vi "例10.8  连续采集图像并保存至avi.vi"() -> ()   [LabVIEW 2017]
doc: "The Grab VI acquires images continuously and displays the images in an image control using high-level acquisition VIs. A grab is appropriate for high-speed applications in which you need to process only one image at a time."
uses:
  <vilib>/userdefined/High Color/IMAQdx.ctl
  <vilib>/vision/driver/NI_Vision_Acquisition_Software.lvlib
panel:
  in  "Frames Per Second":u32=30
  in  "Camera Name":T1
  out "Buffer Number":u32
  out "Image":T2(plugin-control)
  in  "stop":bool
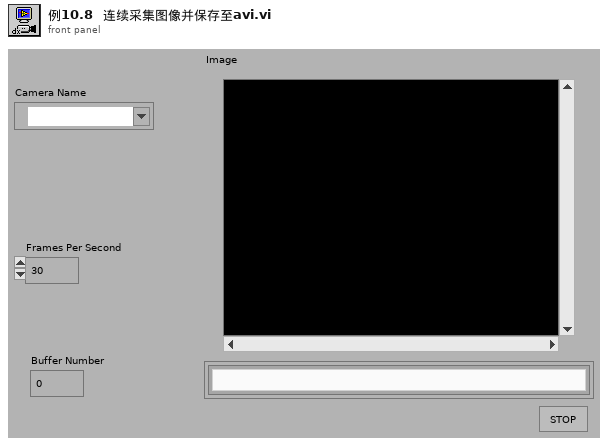
[diagram p1: front panel]
types:
  T1 = typedef "IMAQdx.ctl" = refnum<k21>
  T2 = typedef "IMAQ Image.ctl" = refnum<image>
  T3 = typedef "AviRefnum.ctl" = refnum<k1>
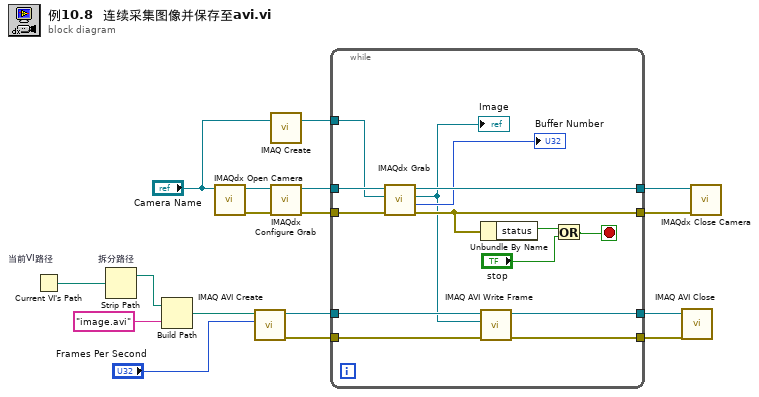
[diagram p0: block diagram]
diagram:
  n1 = Current VI's Path "当前VI路径"() -> (path=w7:path)
  n2 = Strip Path "拆分路径"(path=w7) -> (stripped path=w6:path)  [unwired: 1 out]
  n3 = Build Path ("创建路径")(base path=w6, name or relative path="image.avi") -> (appended path=w5:path)
  n4 = call <vilib>:"IMAQdx Open Camera.vi"("Session In"="Camera Name") -> ("error out"=w12:errorcluster, "Session Out"=w11:T1)  [unwired: 2 in, 7 out]
  n5 = call "IMAQ AVI Create"("Frames Per Second"="Frames Per Second", "AVI Path"=w5) -> ("error out"=w3:errorcluster, "Avi Refnum"=w4:T3)  [unwired: 5 in, 3 out]
  n6 = call "IMAQ Create"("Image Name"="Camera Name") -> ("New Image"=w17:T2)  [unwired: 3 in, 2 out]
  n7 = call <vilib>:"IMAQdx Configure Grab.vi"("error in"=w12, "Session In"=w11) -> ("error out"=w15:errorcluster, "Session Out"=w16:T1)  [unwired: 8 out]
  n8 = while {
    tunnel: [w25] -> w14
    tunnel: w15 -> [w27]
    tunnel: w16 -> [w28]
    tunnel: [w24] -> w13
    tunnel: w17 -> [w26]
    tunnel: w4 -> [w22]
    tunnel: w3 -> [w21]
    tunnel: [w19] -> w2
    tunnel: [w18] -> w1
    stop <- w31 stop-if-true
    n9 = call <vilib>:"IMAQdx Grab.vi"("error in"=w27, "Image In"=w26, "Session In"=w28) -> ("error out"=w24:errorcluster, "Buffer Number Out"=→"Buffer Number":u32, "Image Out"=w20:T2, "Session Out"=w25:T1)  [unwired: 1 in, 4 out]
    "Image" <- w20
    n10 = Unbundle By Name(w24) -> ("status"=w30:bool)
    n11 = call "IMAQ AVI Write Frame"("error in (no error)"=w21, "Image"=w20, "Avi Refnum"=w22) -> ("error out"=w18:errorcluster, "Avi Refnum (duplicate)"=w19:T3)  [unwired: 1 in, 6 out]
    n12 = Or(x=w30, y="stop") -> (x .or. y?=w31:bool)
  }
  n13 = call "IMAQ AVI Close"("error in (no error)"=w1, "Avi Refnum"=w2) -> ()  [unwired: 10 out]
  n14 = call <vilib>:"IMAQdx Close Camera.vi"("error in"=w13, "Session In"=w14) -> ()  [unwired: 10 out]
